vi "test_Set and Get 9437.vi"(8 "error in (no error)":errorcluster, 11 "TestCase in":refnum<class "Scan Engine Scripting API Custom Device Unit Tests.lvclass">) -> (0 "error out":errorcluster, 3 "TestCase out":refnum<class "Scan Engine Scripting API Custom Device Unit Tests.lvclass">)   [LabVIEW 2017, in "Scan Engine Scripting API Custom Device Unit Tests.lvclass"]
uses:
  Scan Engine Scripting API Custom Device Unit Tests.lvclass
  Scan Engine Scripting API Custom Device Unit Tests.lvclass/Scan Engine Scripting API Custom Device Unit Tests.ctl
  6302cd3f-ba9a-4d95-8d24-0299fad587e2.vi
  Utility/Set Error.vi
  <vilib>/Utility/error.llb/Clear Errors.vi
  Scripting/Modules/NI 9437/NI 9437.lvclass
  C:/dev/github.com/debryant/niveristand-scan-engine-ethercat-custom-device/Custom Device Source/Scripting/Modules/Module/Module.lvclass
  Modules.lvlibp/SD Module/SD Module.lvclass
  C:/dev/github.com/debryant/niveristand-scan-engine-ethercat-custom-device/Custom Device Source/Modules.lvlibp/RSI Module/RSI Module.lvclass
  Modules.lvlibp/RSI Module/Read Module Page Property.vi
  Modules.lvlibp/RSI Module/Read Model.vi
  Scripting/Utility/Convert Module Model to Module Class.vi
  Modules.lvlibp/SD Module/Read DIO mode.vi
  Modules.lvlibp/RSI Module/Read Channels.vi
  Scripting/Utility/Convert to DI Module.vi
  Scripting/Utility/Convert to DO Module.vi
  Scripting/Utility/Convert to CI PWM Module.vi
  Scripting/Utility/Convert to CDO Module.vi
  Scripting/Utility/Convert to PWM Module.vi
  Globals/Error Strings.vi
  Scripting/Utility/Convert to AI Vrms Module.vi
  Scripting/Utility/Convert to AI Module.vi
  Scripting/Modules/Module/Module.lvclass
  <vilib>/addons/_JKI Toolkits/VI Tester/TestCase.llb/TestCase.lvclass
  Scripting/Scan Engine Scripting.lvlib
  C:/Program Files (x86)/National Instruments/LabVIEW 2017/vi.lib/addons/_JKI Toolkits/VI Tester/TestCase.llb/TestCase.lvclass
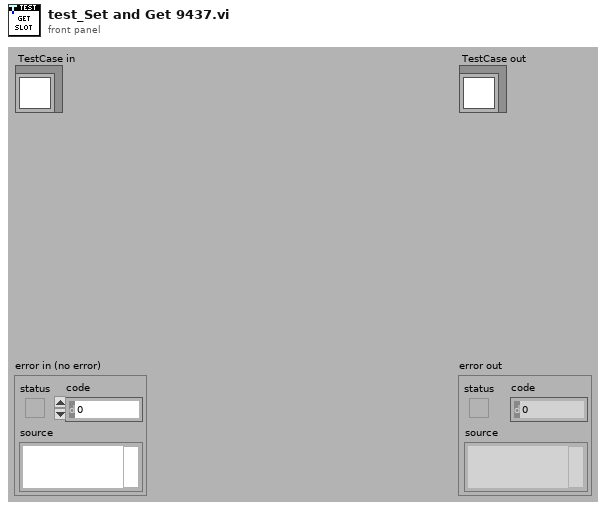
[diagram p1: front panel]
types:
  T1 = typedef "Custom Device API.lvlib/Custom Device Item Ref.ctl" = u64
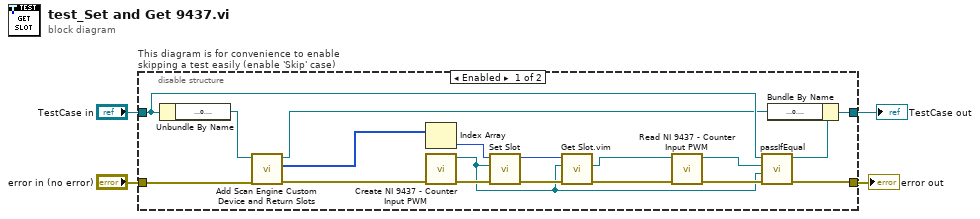
[diagram p0: block diagram]
diagram:
  n1 = disable-structure "This diagram is for convenience to enable skipping a test easily (enable 'Skip' case)" shown="Enabled" {
    disable-tunnel: "TestCase in" -> [w19 w26]
    disable-tunnel: [w21 w24] -> w1
    disable-tunnel: [w17 w25] -> w3
    disable-tunnel: "error in (no error)" -> [w12 w23]
    frame Enabled {
      n2 = Unbundle By Name(w19) -> ("target ref"=w10:refnum<k24>)
      n3 = call "Add Scan Engine Custom Device and Return Slots.vi"("error in"=w12, "target ref in"=w10) -> ("error out"=w11:errorcluster, "slot refs"=w8:T1[], "target ref out"=w9:refnum<k24>)  [unwired: 7 in]
      n4 = Index Array(array=w8) -> (element=w22:T1)  [unwired: 1 in]
      n5 = call "Create NI 9437 - Counter Input PWM.vi"("error in"=w11) -> ("error out"=w18:errorcluster, "NI 9437 out"=w7:refnum<class "NI 9437.lvclass">)  [unwired: 9 in]
      n6 = call "Set Slot.vi"("error in"=w18, "module"=w7, "slot ref in"=w22) -> ("error out"=w20:errorcluster, "slot ref out"=w13:T1)  [unwired: 7 in]
      n7 = call "Get Slot.vim"("error in"=w20, "module in"=w7, "slot ref in"=w13) -> ("error out"=w5:errorcluster, "module"=w6:refnum<class "NI 9437.lvclass">)  [unwired: 5 in, 2 out]
      n8 = call "Read NI 9437 - Counter Input PWM.vi"("error in"=w5, "NI 9437 in"=w6) -> ("error out"=w15:errorcluster, "NI 9437 out"=w16:refnum<class "NI 9437.lvclass">)  [unwired: 7 in, 1 out]
      n9 = call-dynamic "passIfEqual.vi"("error in (no error)"=w15, "y"=w7, "x"=w16, "TestCase in"=w19) -> ("error out"=w17:errorcluster, "TestCase out"=w14:refnum<class "Scan Engine Scripting API Custom Device Unit Tests.lvclass">)  [unwired: 6 in]
      n10 = Bundle By Name(cluster=w14, "target ref"=w9) -> (w21:refnum<class "Scan Engine Scripting API Custom Device Unit Tests.lvclass">)
    }
    frame Disabled {
      # "skip test result while test is under development"
      n11 = call <vilib>:"skip.vi"("error in (no error)"=w23, "TestCase in"=w26) -> ("error out"=w25:errorcluster, "TestCase out"=w24:refnum<class "Scan Engine Scripting API Custom Device Unit Tests.lvclass">)  [unwired: 8 in]
    }
  }
  "error out" <- w3
  "TestCase out" <- w1
